vi "hasStateStored.vi"(8 "error in (no error)":errorcluster, 11 "Client ID":string) -> (0 "error out":errorcluster, 1 "Found?":bool, 2 "Stored Session":T1 {"PUBREC" format="%016b"})   [LabVIEW 2013, in "MQTT Server.lvlib" / "StoredSessions.lvclass"]
uses:
  StoredSessions.lvclass
  Session State -- cluster.ctl
  <vilib>/LabVIEW Open Source Project/MQTT Control Packets/Control Packets/SUBSCRIBE/Topic Subscription -- cluster.ctl
  <vilib>/LabVIEW Open Source Project/MQTT Control Packets/Control Packets/ControlPacket/QualityOfService -- enum.ctl
  <vilib>/LabVIEW Open Source Project/MQTT Control Packets/Control Packets/ControlPacket/ControlPacket.lvclass
  <vilib>/LabVIEW Open Source Project/MQTT Control Packets/Control Packets/SUBSCRIBE/SUBSCRIBE.lvclass
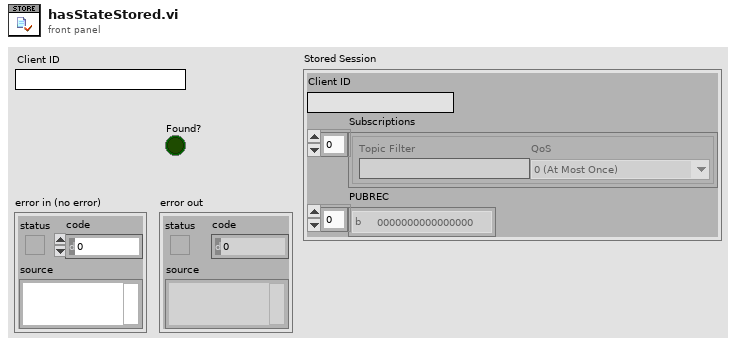
[diagram p1: front panel]
types:
  T1 = typedef "MQTT Server.lvlib/StoredSessions.lvclass/Session State -- cluster.ctl" = cluster{"Client ID":string, "Subscriptions":T2[], "PUBREC":u16[]}
  T2 = typedef "MQTT_Control_Packets.lvlib/SUBSCRIBE.lvclass/Topic Subscription -- cluster.ctl" = cluster{"Topic Filter":string, "QoS":T3}
  T3 = typedef "MQTT_Control_Packets.lvlib/ControlPacket.lvclass/QualityOfService -- enum.ctl" = enum16{"0 (At Most Once)", "1 (At Least Once)", "2 (Exactly Once)"}
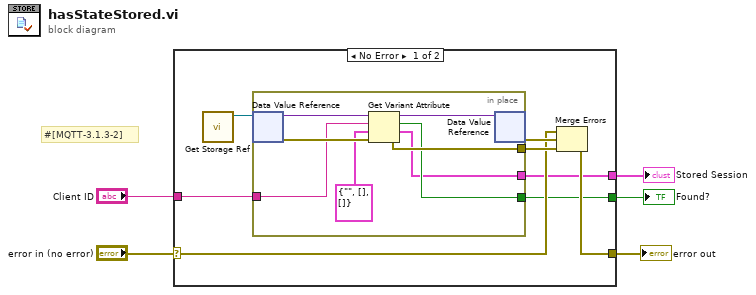
[diagram p0: block diagram]
diagram:
  # "#[MQTT-3.1.3-2]"
  n1 = case shown="No Error" "error in (no error)" {
    selector: "error in (no error)" -> [w9 w22]
    tunnel: [w8 w22] -> w4
    tunnel: "Client ID" -> [w12 _]
    tunnel: [w7 _] -> w2
    tunnel: [w6 _] -> w1
    frame No Error {
      n2 = call "Get Storage Ref.vi"() -> ("Storage"=w13:refnum<data-value>)  [unwired: 11 in]
      n3 = in-place {
        in-place-border: w12 -> [w17]
        in-place-border: [w20] -> w11
        in-place-border: [w16] -> w7
        in-place-border: [w15] -> w6
        n4 = in-place-dvr #1(w13) -> (w18:variant, w19:errorcluster)
        n5 = Get Variant Attribute(Variant=w18, name=w17, default value (empty Variant)=T1 {"Client ID"="", "Subscriptions"=[], "PUBREC"=[]} ("Stored Session"), error in=w19) -> (duplicate Variant=w21:variant, found=w16:bool, value=w15:T1, error out=w20:errorcluster)
        n6 = in-place-dvr #1(w21) -> (w10:errorcluster)  [unwired: 1 out]
      }
      n7 = Merge Errors(w9, w10, w11) -> (w8:errorcluster)
    }
    frame Error {
    }
  }
  "error out" <- w4
  "Found?" <- w2
  "Stored Session" <- w1
